vi "Configure Current Limit.vi"(8 "error in (no error)":errorcluster, 9 "Current Limit (0.0 A)":dbl format="%.2g", 11 "VISA resource name":refnum<visa-resource-name>) -> (0 "error out":errorcluster, 3 "VISA resource name out":refnum<visa-resource-name>)   [LabVIEW 2022 SP3, in "BK Precision 9103.lvlib"]
doc: "Configures over current protection (OCP). Specify the output current limit value and the behavior of the power supply when the output current is greater than or equal to that value."
uses:
  <instrlib>/BK Precision 9103/BK Precision 9103.lvlib
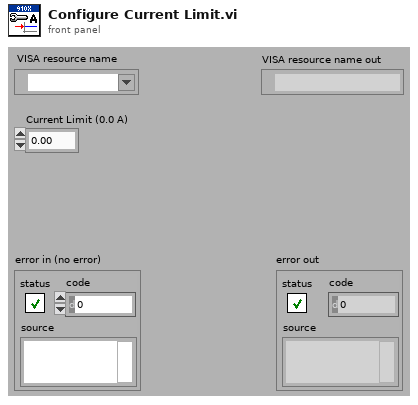
[diagram p1: front panel]
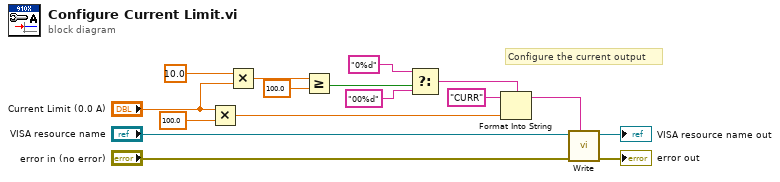
[diagram p0: block diagram]
diagram:
  # "Configure the current output"
  n1 = Multiply(x="Current Limit (0.0 A)", y=100.0) -> (x*y=w7:dbl)
  n2 = Multiply(x=10.0 ("y"), y="Current Limit (0.0 A)") -> (x*y=w15:dbl)
  n3 = Greater Or Equal?(x=w15, y=100.0) -> (x >= y?=w13:bool)
  n4 = Select(t="0%d" ("format string"), s=w13, f="00%d" ("format string")) -> (s? t:f=w9:string)
  n5 = Format Into String(format string=w9, initial string="CURR", w7) -> (resulting string=w1:string)  [unwired: 1 in, 1 out]
  n6 = call <instrlib>:"Write.vi"("Input String"=w1, "error in (no error)"="error in (no error)", "VISA resource name"="VISA resource name") -> ("error out"=→"error out":errorcluster, "VISA resource name out"=→"VISA resource name out":refnum<visa-resource-name>)  [unwired: 7 in]
